vi "GetReportsList(SubVI).vi"(8 "error in (no error)":errorcluster) -> (0 "error out":errorcluster, 3 "Available Reports":string[](array[string]))   [LabVIEW 2017, in "MainFrameLib.lvlib"]
uses:
  MainFrameLib.lvlib
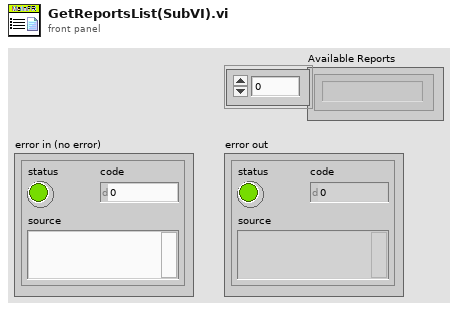
[diagram p1: front panel]
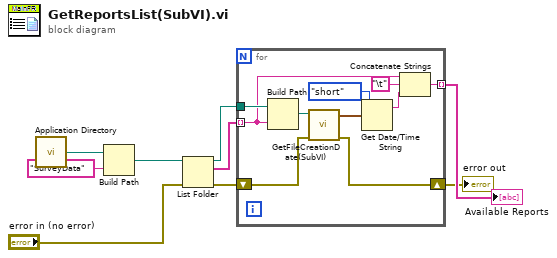
[diagram p0: block diagram]
diagram:
  n1 = call <vilib>:"Application Directory.vi"() -> ("Application Directory"=w2:path)
  n2 = Build Path(base path=w2, name or relative path="SurveyData") -> (appended path=w4:path)
  n3 = List Folder(path=w4, error in="error in (no error)") -> (path out=w5:path, filenames=w7:string[], error out=w6:errorcluster)  [unwired: 2 in, 1 out]
  n4 = for {
    tunnel: w5 -> [w19]
    tunnel: w7 -> [w11] mode=indexing
    shift-right: [w16] -> w8
    shift-left: w6 -> [w17]
    tunnel: [w10] -> w9 mode=indexing
    n5 = Build Path(base path=w19, name or relative path=w11) -> (appended path=w18:path)
    n6 = call "GetFileCreationDate(SubVI).vi"("Error In"=w17, "File Path"=w18) -> ("Error Out"=w16:errorcluster, "File Created Date (UTC)"=w15:timestamp)  [unwired: 6 in]
    n7 = Get Date/Time String(date format (0)=enum16{"short", "long", "abbreviated"}."short", seconds (now)=w15) -> (date string=w13:string)  [unwired: 1 in, 1 out]
    n8 = Concatenate Strings(w11, "\t", w13) -> (w10:string)
  }
  "Available Reports" <- w9
  "error out" <- w8
